vi "SetCursorPosition.vi"(11 "XY":cluster{"X":dbl, "Y":dbl}) -> ()   [LabVIEW 2013, in "main.lvlib"]
uses:
  main.lvlib
  USER32.DLL
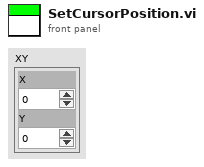
[diagram p1: front panel]
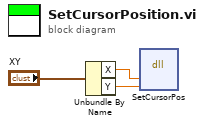
[diagram p0: block diagram]
diagram:
  n1 = Unbundle By Name("XY") -> ("X"=w1:dbl, "Y"=w2:dbl)
  n2 = dll-call lib="user32.dll" fn="SetCursorPos"("dx"=w1, "dy"=w2) -> ()  [unwired: 6 in, 2 out]
